vi "Main2.vi"() -> ()   [LabVIEW 2014]
doc: "Use this template to build a simple state machine design pattern. Each state executes code and determines which state to transition to."
uses:
  controls/State.ctl
  controls/Data.ctl
  Program Files/National Instruments/LabVIEW 2013/examples/Instrument IO/Serial/support/Serial - Settings.ctl
panel:
  out "Data":T1
  in  "Exit":bool
  # "This template is for the Simple State Machine design pattern.\n\nSee the block diagram for more information on how to use this template."
  # "These controls have associated \"Value Changed\" events configured in the Event Structure on the diagram.\n\nReplace them (and reconfigure the Event Structure) with the controls you need for your application."
  # "日期"
  # "機種名稱"
  # "機種代號"
  # "商品條碼"
  # "台"
  # "OK"
  # "NG"
  # "台"
  # "總計"
  # "台"
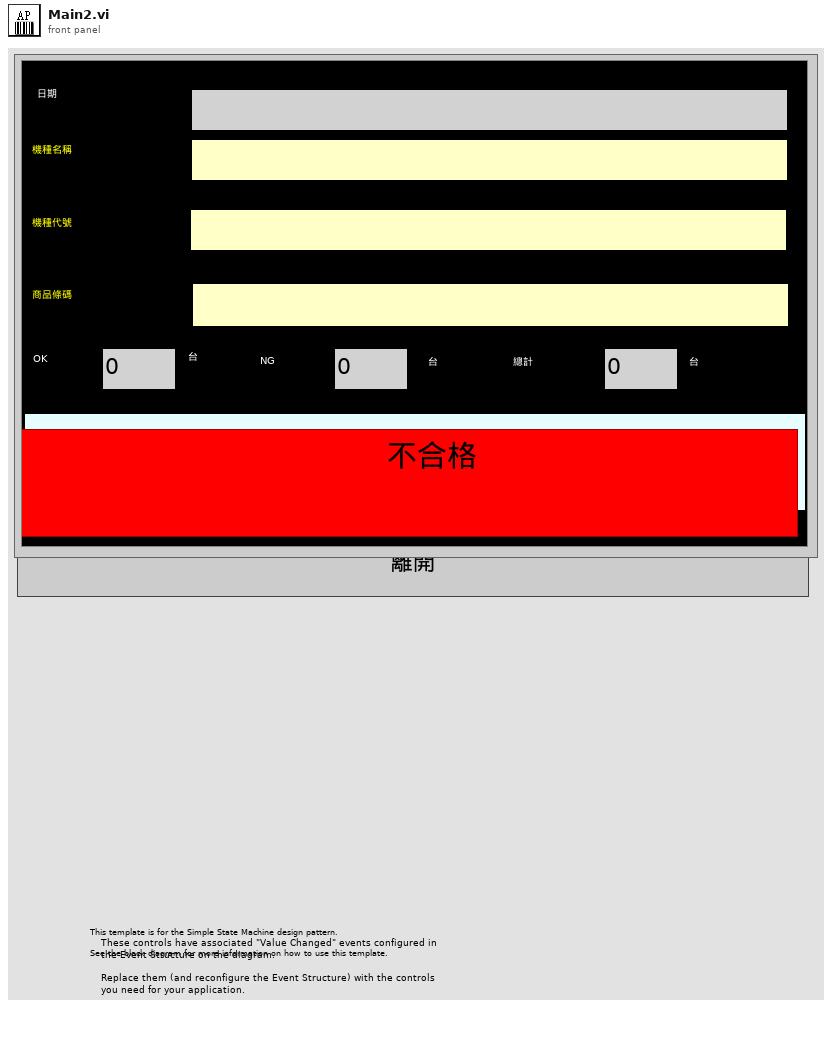
[diagram p1: front panel]
types:
  T1 = typedef "Data.ctl" = cluster{"Date":string, "BarCode1":string, "BarCode2":string, "BarCode3":string, "Message":string, "OK Count":u16, "NG Count":u16, "Total Count":u16, "ModelData":string[][], "OK&NG":bool, "COM1":refnum<visa-resource-name>, "COM2":refnum<visa-resource-name>, "IO":i32, "Time":u32, "TCP":refnum<k5>, "TCP 2":refnum<k5>}
  T2 = typedef "State.ctl" = enum16{"Initialize", "Wait for Scan", "State 1", "State 2", "NG", "NG1", "OK", "OKNG", "Exit"}
  T3 = typedef "Serial - Settings.ctl" = cluster{"baud rate":u32, "data bits":u16, "parity":enum16{"None", "Odd", "Even", "Mark", "Space"}, "stop bits":u16, "flow control":u16}
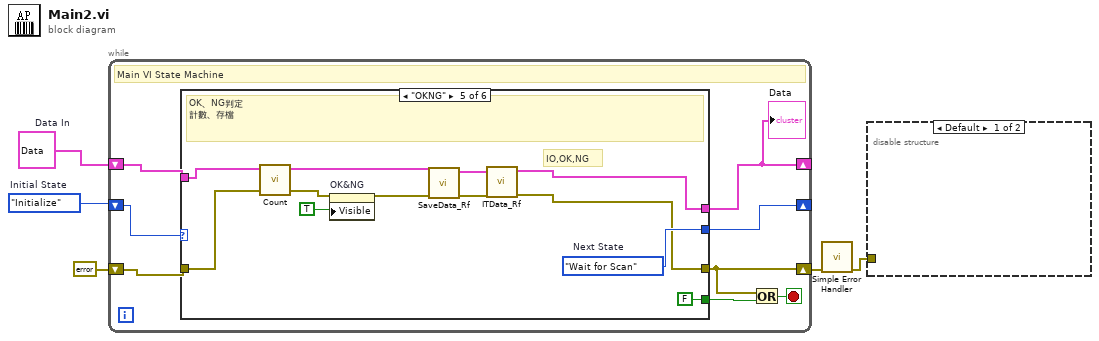
[diagram p0: block diagram]
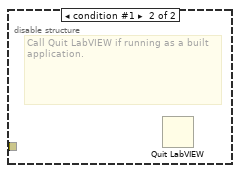
[diagram p2: hidden frame]
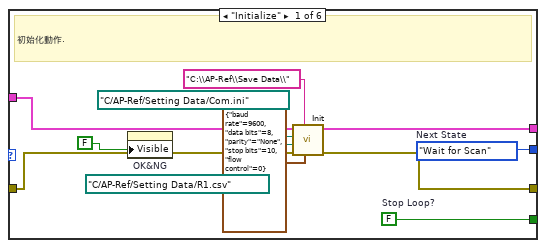
[diagram p3: hidden frame]
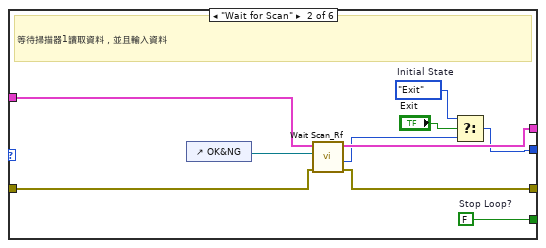
[diagram p4: hidden frame]
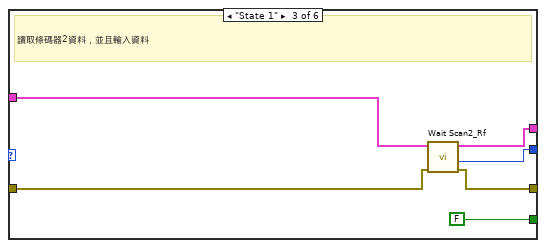
[diagram p5: hidden frame]
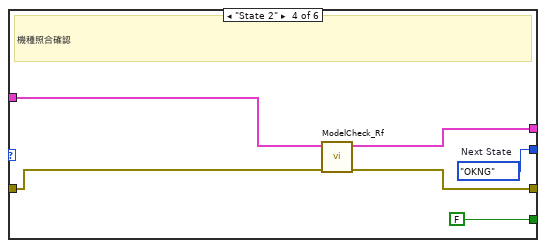
[diagram p6: hidden frame]
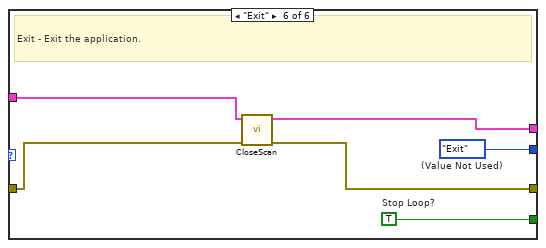
[diagram p7: hidden frame]
diagram:
  w1 = T1 {"Date"="", "BarCode1"="", "BarCode2"="", "BarCode3"="", "Message"="", "OK Count"=0, "NG Count"=0, "Total Count"=0, "ModelData"=[], "OK&NG"=FALSE, "COM1"="", "COM2"="", "IO"=0, "Time"=0, "TCP"=refnum, "TCP 2"=refnum}  # Data In
  w2 = State."Initialize"  # Initial State
  n1 = while {
    shift-right: [w10] -> _
    shift-left: w2 -> [w8]
    shift-right: [w6] -> _
    shift-left: w1 -> [w11]
    shift-right: [w7] -> w4
    shift-left: errorcluster {"status"=FALSE, "code"=0, "source"=""} ("error constant") -> [w9]
    stop <- w12 stop-if-true
    # "Main VI State Machine"
    n2 = case shown="\"OKNG\"" w8 {
      tunnel: [w24 w34 FALSE ("Stop Loop?") FALSE ("Stop Loop?") FALSE ("Stop Loop?") w63] -> w13
      tunnel: w9 -> [w20 w28 w37 w42 w48 w59]
      tunnel: [w19 w27 w36 w41 w50 w58] -> w7
      tunnel: w11 -> [w23 w33 w39 w45 w55 w61]
      tunnel: [w22 w32 w38 w43 w51 w60] -> w6
      tunnel: [w21 w26 w35 w44 w54 w62] -> w10
      frame "Initialize" {
        w24 = FALSE  # Stop Loop?
        w21 = State."Wait for Scan"  # Next State
        # "初始化動作."
        n3 = property on="OK&NG" class="Bool (strict)"("Visible"=FALSE) -> ()  [unwired: 2 in, 2 out]
        n4 = call "Init.vi"(6:T3 {"baud rate"=9600, "data bits"=8, "parity"=enum."None", "stop bits"=10, "flow control"=0} ("Serial Settings"), "Save Path"="C:\\AP-Ref\\Save Data\\", "error in (no error)"=w20, "Model Path"=path "C:/AP-Ref/Setting Data/R1.csv", "IO Path"=path "C:/AP-Ref/Setting Data/Com.ini", "Data In"=w23) -> ("error out"=w19:errorcluster, "Data Out"=w22:T1)  [unwired: 4 in]
      }
      frame "Wait for Scan" {
        w30 = State."Exit"  # Initial State
        w34 = FALSE  # Stop Loop?
        # "等待掃描器1讀取資料，並且輸入資料"
        n5 = control-ref of="OK&NG"() -> (w25:refnum<vi>)
        n6 = call "Wait Scan_Rf.vi"("error in (no error)"=w28, "OK&NG"=w25, "Data In"=w33) -> ("error out"=w27:errorcluster, "States"=w29:T2, "Data Out"=w32:T1)  [unwired: 6 in]
        n7 = Select(t=w30, s="Exit", f=w29) -> (s? t:f=w26:T2)
      }
      frame "State 1" {
        # "讀取條碼器2資料，並且輸入資料"
        n8 = call "Wait Scan2_Rf.vi"("error in (no error)"=w37, "Data In"=w39) -> ("error out"=w36:errorcluster, "States"=w35:T2, "Data Out"=w38:T1)  [unwired: 7 in]
      }
      frame "State 2" {
        w44 = State."OKNG"  # Next State
        # "機種照合確認"
        n9 = call "ModelCheck_Rf.vi"("error in (no error)"=w42, "Data In"=w45) -> ("error out"=w41:errorcluster, "Data Out"=w43:T1)  [unwired: 8 in]
      }
      frame "OKNG" {
        w54 = State."Wait for Scan"  # Next State
        # "IO,OK,NG"
        # "OK、NG判定\n計數、存檔"
        n10 = call "Count.vi"("Data In"=w55) -> ("Data Out"=w57:T1)  [unwired: 10 in]
        n11 = property on="OK&NG" class="Bool (strict)"(error in=w48, "Visible"=TRUE) -> (error out=w47:errorcluster)  [unwired: 1 in, 1 out]
        n12 = call "SaveData_Rf.vi"("error in (no error)"=w47, "Data In"=w57) -> ("error out"=w52:errorcluster, "Data Out"=w53:T1)  [unwired: 8 in]
        n13 = call "ITData_Rf.vi"("error in (no error)"=w52, "Data In"=w53) -> ("error out"=w50:errorcluster, "Data Out"=w51:T1)  [unwired: 8 in]
      }
      frame "Exit" {
        w63 = TRUE  # Stop Loop?
        w62 = State."Exit"  # (Value Not Used)
        # "Exit - Exit the application."
        n14 = call "CloseScan.vi"("error in (no error)"=w59, "Data In"=w61) -> ("error out"=w58:errorcluster, "Data Out"=w60:T1)  [unwired: 8 in]
      }
    }
    "Data" <- w6
    n15 = Or(x=w7, y=w13) -> (x .or. y?=w12:bool)
  }
  n16 = call <vilib>:"Simple Error Handler.vi"("error in (no error)"=w4) -> ("error out"=w3:errorcluster)  [unwired: 4 in, 4 out]
  n17 = disable-structure shown="Default" {
    disable-tunnel: w3 -> [_ _]
    frame condition #0 (active) {
    }
    frame condition #1 {
      # "Call Quit LabVIEW if running as a built application."
      n18 = Quit LabVIEW() -> ()  [unwired: 1 in]
    }
  }
